vi "AC-Transfer.vi"() -> ()   [LabVIEW 2014]
uses:
  <vilib>/Analysis/4window.llb/windowTd.ctl
  <vilib>/DAQmx/configure/timing.llb/DAQmx Timing (Sample Clock).vi
  <vilib>/DAQmx/read.llb/DAQmx Read (Analog 2D DBL NChan NSamp).vi
  <vilib>/DAQmx/write.llb/DAQmx Write (Analog Wfm 1Chan NSamp).vi
  <vilib>/Analysis/1siggen.llb/Ramp Pattern by Samples.vi
  <vilib>/measure/maspectr.llb/FFT Power Spectrum and PSD for 1 Chan.vi
  <vilib>/DAQmx/configure/trigger.llb/DAQmx Start Trigger (Digital Edge).vi
  <vilib>/DAQmx/create/channels.llb/DAQmx Create Channel (AI-Voltage-Basic).vi
  <vilib>/measure/maspectr.llb/Frequency Response Function (Mag-Phase) 1-1.vi
  <vilib>/DAQmx/create/channels.llb/DAQmx Create Channel (AO-Voltage-Basic).vi
  <vilib>/Utility/file.llb/Write To Spreadsheet File (DBL).vi
  <resource>/objmgr/daqmx.rc
  <vilib>/measure/NI_MABase.lvlib
  <vilib>/Analysis/NI_AALBase.lvlib
  <vilib>/measure/NI_MAPro.lvlib
  <vilib>/Analysis/NI_AALPro.lvlib
panel:
  out "Phase response":cluster{dbl[], dbl[]}(graph)
  out "Magnitude response":cluster{dbl[], dbl[]}(graph)
  out "Actual Freq [Hz]":dbl format="%#_6p"
  out "Measured signals":waveform(dbl)[](graph)
  in  "Sweep poins":i32=30
  in  "Sweep end [Hz]":dbl=1000.0
  in  "Sweep start [Hz]":dbl=1.0
  in  "Amplitude":dbl=1.0
  out "Actual Fs [Hz]":dbl
  in  "Sampling freq [Hz]":dbl=100000.0 format="%#_6p"
  in  "Sampled points":i32=65536
  in  "Trigger Source (ai/StartTrigger)":tag="/cDAQ2/ai/StartTrigger"
  in  "Output Channel (Mod2/ao1)":tag="cDAQ2Mod2/ao0"
  in  "Input Channels (Mod1/ai0:1)":tag="cDAQ2Mod1/ai0:1"
  # "Channel Settings"
  # "Measurement settings"
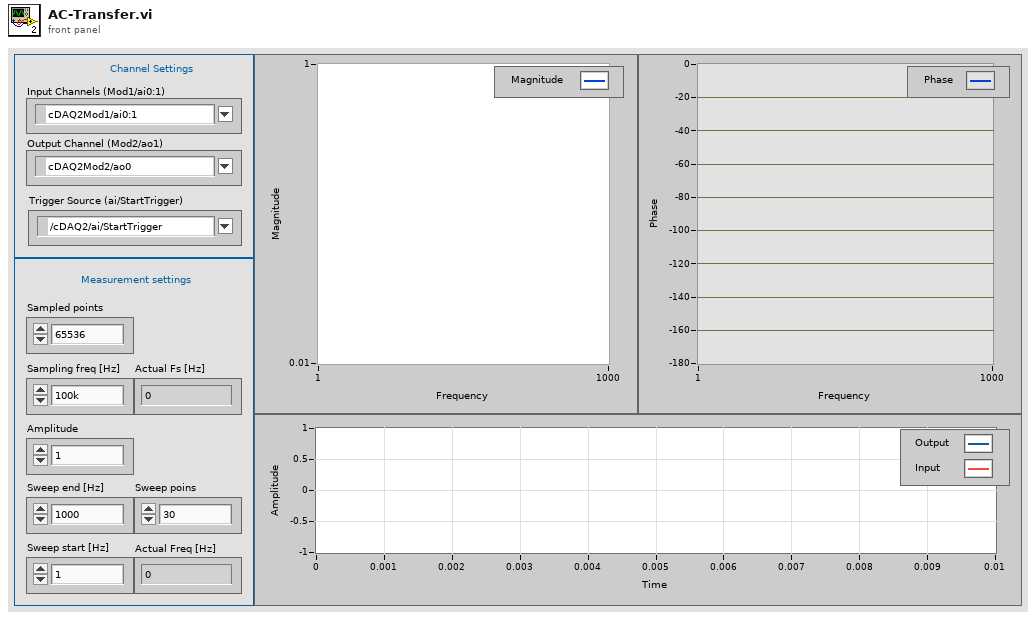
[diagram p1: front panel]
types:
  T1 = typedef "NI_AALPro.lvlib/windowTd.ctl" = u32
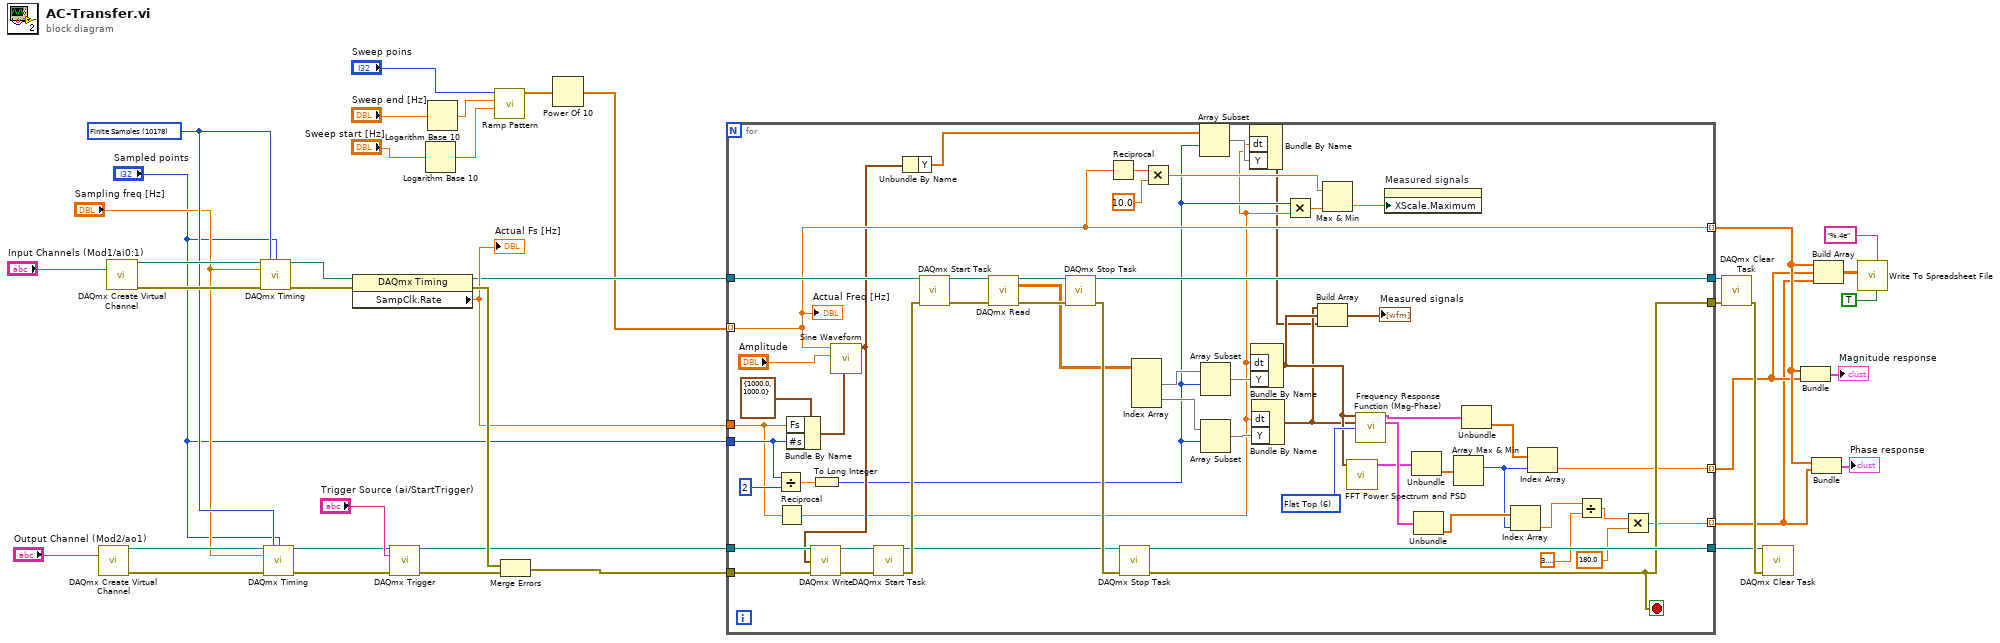
[diagram p0: block diagram]
diagram:
  w32 = 10178 items=["Finite Samples"=10178, "Continuous Samples"=10123, "Hardware Timed Single Point"=12522] ("sample mode")
  n1 = call-poly <vilib>:"DAQmx Create Virtual Channel.vi"("physical channels"="Output Channel (Mod2/ao1)") -> ("task out"=w38:refnum<k21>, "error out"=w36:errorcluster)  [unwired: 13 in]
  n2 = call-poly <vilib>:"DAQmx Create Virtual Channel.vi"("physical channels"="Input Channels (Mod1/ai0:1)") -> ("task out"=w39:refnum<k21>, "error out"=w37:errorcluster)  [unwired: 13 in]
  n3 = call-poly <vilib>:"DAQmx Timing.vi"("task/channels in"=w39, "sample mode"=w32, "samples per channel"="Sampled points", "rate"="Sampling freq [Hz]", "error in"=w37) -> ("task out"=w35:refnum<k21>, "error out"=w34:errorcluster)  [unwired: 9 in]
  n4 = call-poly <vilib>:"DAQmx Timing.vi"("task/channels in"=w38, "sample mode"=w32, "samples per channel"="Sampled points", "rate"="Sampling freq [Hz]", "error in"=w36) -> ("task out"=w7:refnum<k21>, "error out"=w33:errorcluster)  [unwired: 9 in]
  n5 = property class="DAQmx Timing"(reference=w35, error in=w34) -> (reference out=w20:refnum<k21>, error out=w28:errorcluster, "SampClk.Rate"=w25:dbl)
  "Actual Fs [Hz]" <- w25
  n6 = call-poly <vilib>:"DAQmx Trigger.vi"("task/channels in"=w7, "source"="Trigger Source (ai/StartTrigger)", "error in"=w33) -> ("task out"=w21:refnum<k21>, "error out"=w27:errorcluster)  [unwired: 11 in]
  n7 = Logarithm Base 10(1:"Sweep start [Hz]") -> (0:w9:dbl)
  n8 = Logarithm Base 10(1:"Sweep end [Hz]") -> (0:w11:dbl)
  n9 = call-poly <vilib>:"Ramp Pattern.vi"("start"=w9, "end"=w11, "samples"="Sweep poins") -> ("Ramp Pattern"=w13:dbl[])  [unwired: 7 in, 1 out]
  n10 = Merge Errors(w28, w27) -> (w22:errorcluster)
  n11 = Power Of 10(x=w13) -> (10^x=w12:dbl[])
  n12 = for {
    tunnel: w25 -> [w69]
    tunnel: "Sampled points" -> [w74]
    tunnel: w12 -> [w51] mode=indexing
    tunnel: w22 -> [w91]
    tunnel: w21 -> [w90]
    tunnel: w20 -> [w85]
    tunnel: [w78] -> w18
    tunnel: [w82] -> w19
    tunnel: [w79] -> w16
    tunnel: [w59] -> w5 mode=indexing
    tunnel: [w54] -> w4 mode=indexing
    tunnel: [w51] -> w6 mode=indexing
    stop <- w78 stop-if-true
    w64 = T1 6 items=["Rectangle"=0, "Hanning"=1, "Hamming"=2, "Blackman-Harris"=3, "Exact Blackman"=4, "Blackman"=5, "Flat Top"=6, "4 Term B-Harris "=7, "7 Term B-Harris"=8, "Low Sidelobe"=9, "Blackman Nuttall"=11, "Triangle"=30, "Bartlett-Hanning"=31, "Bohman"=32, "Parzen"=33, "Welch"=34, "Kaiser"=60, "Dolph-Chebyshev"=61, "Gaussian"=62] ("window")
    n13 = Divide(x=w74, y=2) -> (x/y=w72:dbl)
    n14 = Reciprocal(x=w69) -> (1/x=w41:dbl)
    n15 = Bundle By Name(cluster=cluster{"Fs":dbl, "#s":dbl} {"Fs"=1000.0, "#s"=1000.0} ("sampling info"), "Fs"=w69, "#s"=w74) -> (w95:cluster{"Fs":dbl, "#s":dbl})
    n16 = To Long Integer(number=w72) -> (32bit integer=w43:i32)
    n17 = call <vilib>:"Sine Waveform.vi"("sampling info"=w95, "amplitude"="Amplitude", "frequency"=w51) -> ("signal out"=w45:waveform(dbl))  [unwired: 7 in, 1 out]
    n18 = call-poly <vilib>:"DAQmx Write.vi"("task/channels in"=w90, "data"=w45, "error in"=w91) -> ("task out"=w89:refnum<k21>, "error out"=w92:errorcluster)  [unwired: 10 in, 1 out]
    n19 = call <vilib>:"DAQmx Start Task.vi"("task/channels in"=w89, "error in"=w92) -> ("task out"=w80:refnum<k21>, "error out"=w86:errorcluster)  [unwired: 12 in]
    n20 = Unbundle By Name(w45) -> ("Y"=w44:dbl[])
    n21 = call <vilib>:"DAQmx Start Task.vi"("task/channels in"=w85, "error in"=w86) -> ("task out"=w88:refnum<k21>, "error out"=w87:errorcluster)  [unwired: 12 in]
    n22 = call-poly <vilib>:"DAQmx Read.vi"("task/channels in"=w88, "error in"=w87) -> ("task out"=w84:refnum<k21>, "data"=w77:dbl[][], "error out"=w83:errorcluster)  [unwired: 11 in]
    n23 = call <vilib>:"DAQmx Stop Task.vi"("task/channels in"=w84, "error in"=w83) -> ("task out"=w82:refnum<k21>, "error out"=w81:errorcluster)  [unwired: 12 in]
    n24 = Reciprocal(x=w51) -> (1/x=w50:dbl)
    n25 = call <vilib>:"DAQmx Stop Task.vi"("task/channels in"=w80, "error in"=w81) -> ("task out"=w79:refnum<k21>, "error out"=w78:errorcluster)  [unwired: 12 in]
    n26 = Index Array(array=w77) -> (element #1=w76:dbl[], element #2=w75:dbl[])  [unwired: 4 in]
    n27 = Multiply(x=w50, y=10.0) -> (x*y=w47:dbl)
    n28 = Array Subset(array=w44, index=w43) -> (w42:dbl[])  [unwired: 1 in]
    n29 = Array Subset(array=w76, index=w43) -> (w71:dbl[])  [unwired: 1 in]
    n30 = Array Subset(array=w75, index=w43) -> (w70:dbl[])  [unwired: 1 in]
    n31 = Bundle By Name("dt"=w41, "Y"=w42) -> (w40:waveform(dbl))  [unwired: 1 in]
    n32 = Bundle By Name("dt"=w41, "Y"=w71) -> (w53:waveform(dbl))  [unwired: 1 in]
    n33 = Bundle By Name("dt"=w41, "Y"=w70) -> (w52:waveform(dbl))  [unwired: 1 in]
    n34 = Multiply(x=w43, y=w41) -> (x*y=w48:dbl)
    n35 = Build Array(w52, w53, w40) -> (→"Measured signals":waveform(dbl)[])
    n36 = Max & Min(x=w47, y=w48) -> (min(x,y)=w46:dbl)  [unwired: 1 out]
    n37 = call-poly <vilib>:"FFT Power Spectrum and PSD.vi"("time signal"=w53) -> ("Power Spectrum / PSD"=w63:cluster{"f0":dbl, "df":dbl, "magnitude":dbl[]})  [unwired: 7 in, 3 out]
    n38 = call-poly <vilib>:"Frequency Response Function (Mag-Phase).vi"("time signal X"=w53, "time signal Y"=w52, "window"=w64) -> ("magnitude"=w62:cluster{"f0":dbl, "df":dbl, "magnitude":dbl[]}, "phase"=w65:cluster{"f0":dbl, "df":dbl, "phase":dbl[]})  [unwired: 7 in, 4 out]
    n39 = property on="Measured signals" class="WFGraph (strict)"("XScale.Maximum"=w46) -> ()  [unwired: 2 in, 2 out]
    n40 = Unbundle(w63) -> ("magnitude"=w67:dbl[])  [unwired: 2 out]
    n41 = Unbundle(w65) -> ("phase"=w66:dbl[])  [unwired: 2 out]
    n42 = Array Max & Min(array=w67) -> (max index (indices)=w60:i32)  [unwired: 3 out]
    n43 = Unbundle(w62) -> ("magnitude"=w61:dbl[])  [unwired: 2 out]
    n44 = Index Array(array=w66, index=w60) -> (element=w58:dbl)
    n45 = Index Array(array=w61, index=w60) -> (element=w59:dbl)
    n46 = Divide(x=w58, y=3.141592653589793) -> (x/y=w56:dbl)
    n47 = Multiply(x=w56, y=180.0) -> (x*y=w54:dbl)
    "Actual Freq [Hz]" <- w51
  }
  n48 = call <vilib>:"DAQmx Clear Task.vi"("task in"=w19, "error in"=w18) -> ("error out"=w17:errorcluster)  [unwired: 13 in]
  n49 = call <vilib>:"DAQmx Clear Task.vi"("task in"=w16, "error in"=w17) -> ()  [unwired: 13 in, 1 out]
  n50 = Bundle(w6, w5) -> (→"Magnitude response":cluster{dbl[], dbl[]})  [unwired: 1 in]
  n51 = Bundle(w6, w4) -> (→"Phase response":cluster{dbl[], dbl[]})  [unwired: 1 in]
  n52 = Build Array(w6, w5, w4) -> (w3:dbl[][])
  n53 = call-poly <vilib>:"Write To Spreadsheet File.vi"("transpose? (no:F)"=TRUE, "format (%.3f)"="%.4e", "2D data"=w3) -> ()  [unwired: 5 in, 1 out]
